vi "DecimateWaveform.vi"(10 "Decimating factor":dbl, 11 "waveform in":waveform(dbl)) -> (2 "Y":dbl[](array[numeric]), 3 "waveform out":waveform(dbl))   [LabVIEW 2017, in "Scope.lvlib"]
uses:
  Scope.lvlib
  <vilib>/Analysis/2dsp.llb/Decimate (single shot, DBL).vi
  <vilib>/Analysis/NI_AALPro.lvlib
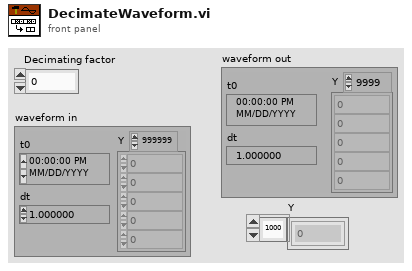
[diagram p1: front panel]
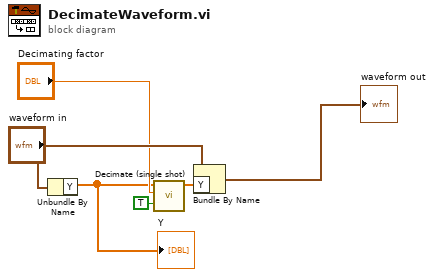
[diagram p0: block diagram]
diagram:
  n1 = Unbundle By Name("waveform in") -> ("Y"=w1:dbl[])
  "Y" <- w1
  n2 = call-poly <vilib>:"Decimate (single shot).vi"("averaging"=TRUE, "decimating factor"="Decimating factor", "X"=w1) -> ("Decimated Array"=w4:dbl[])  [unwired: 7 in, 1 out]
  n3 = Bundle By Name(cluster="waveform in", "Y"=w4) -> (→"waveform out":waveform(dbl))
